vi "dummyTriggerVIref.vi"() -> ()   [LabVIEW 2019]
panel:
  in  "VI Refnum":refnum<vi>
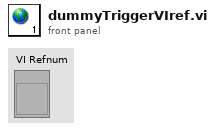
[diagram p1: front panel]
diagram:
